vi "RP100 ini.vi"(7 "Error Queue Option":enum16{"Clear Error Queue", "Error Query"}(ring), 8 "error in (no error)":errorcluster, 9 "ID Query? (T)":bool, 10 "Reset? (T)":bool, 11 "VISA resource name":refnum<visa-resource-name>) -> (0 "error out":errorcluster, 3 "VISA resource name out":refnum<visa-resource-name>)   [LabVIEW 2019, in "RP100.lvlib"]
uses:
  RP100.lvlib
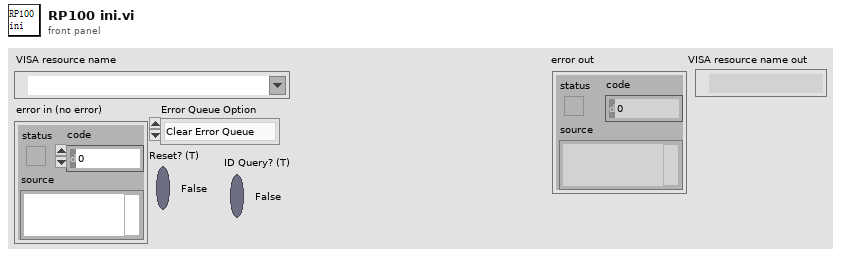
[diagram p1: front panel]
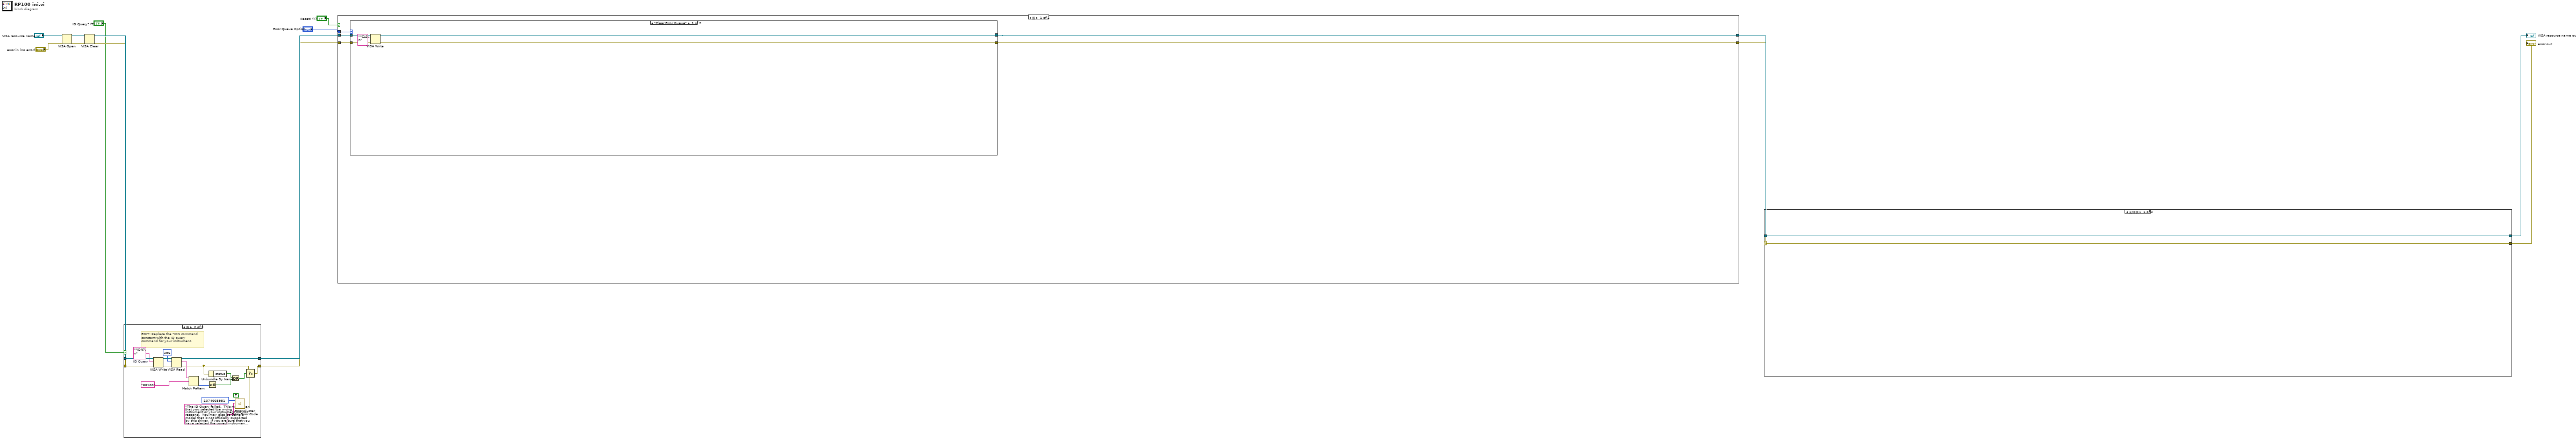
[diagram p0: block diagram]
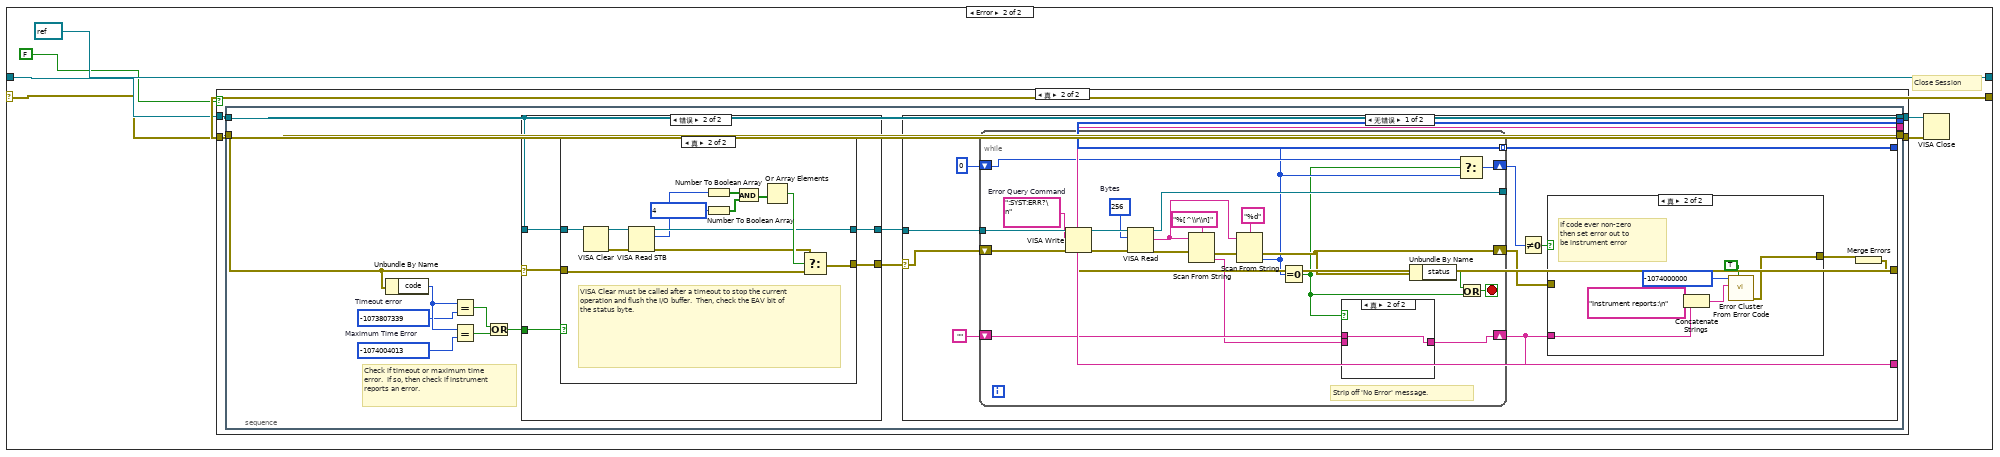
[diagram p2: hidden frame]
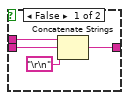
[diagram p7: hidden frame]
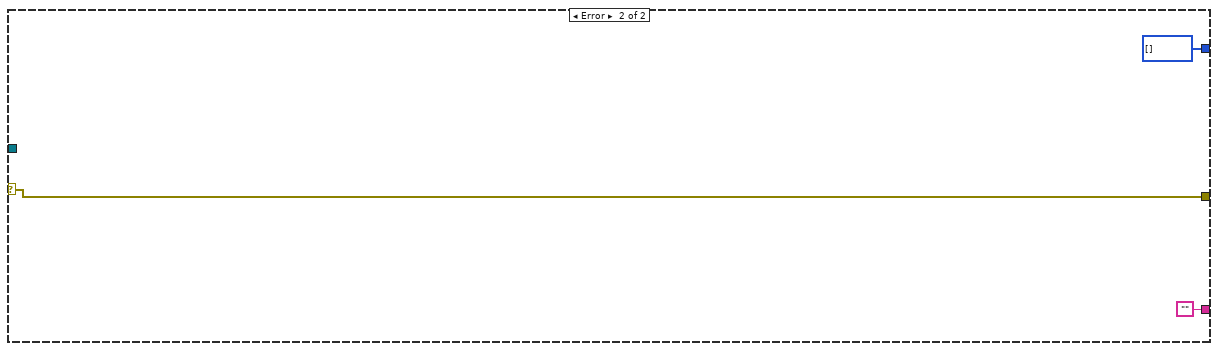
[diagram p8: hidden frame]
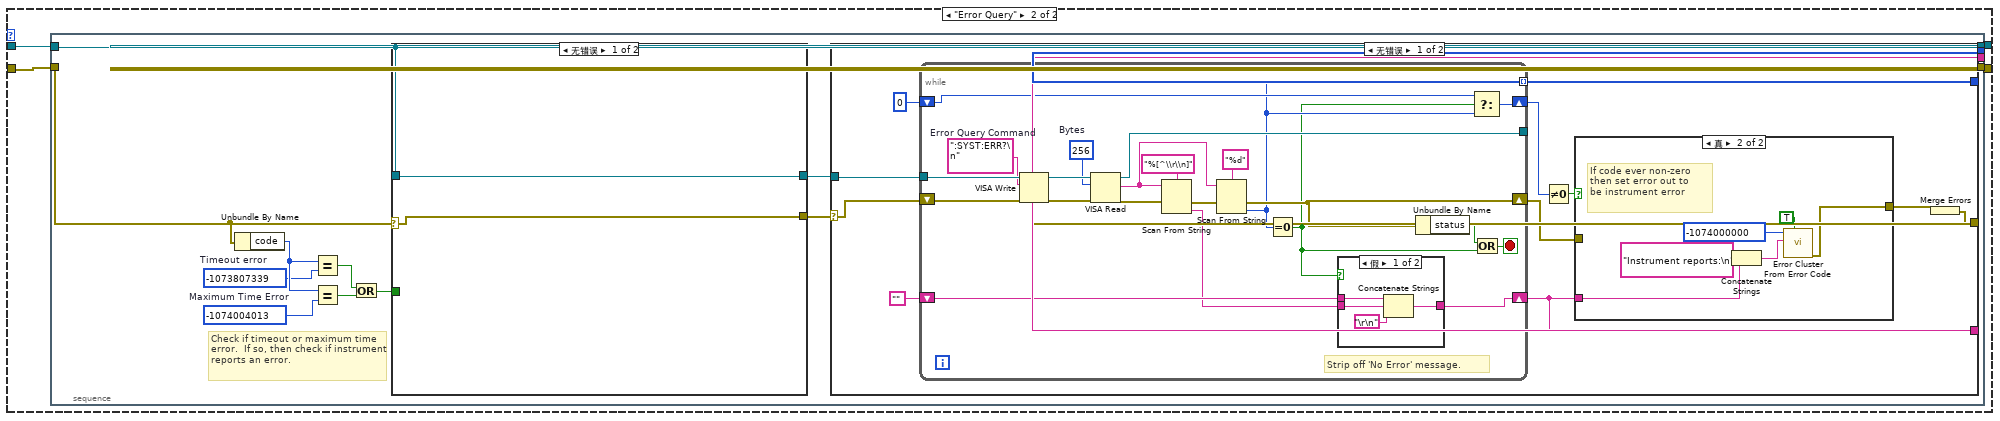
[diagram p9: hidden frame]
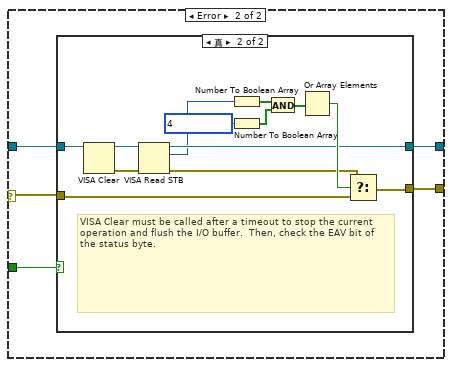
[diagram p10: hidden frame]
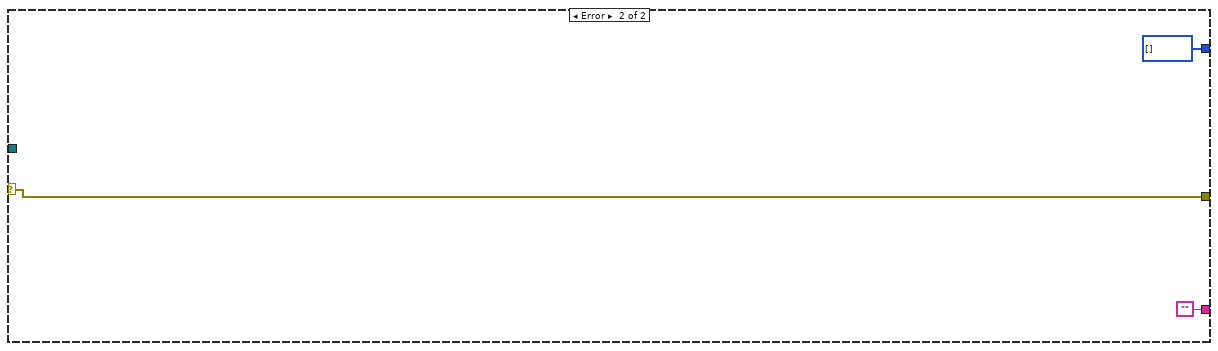
[diagram p14: hidden frame]
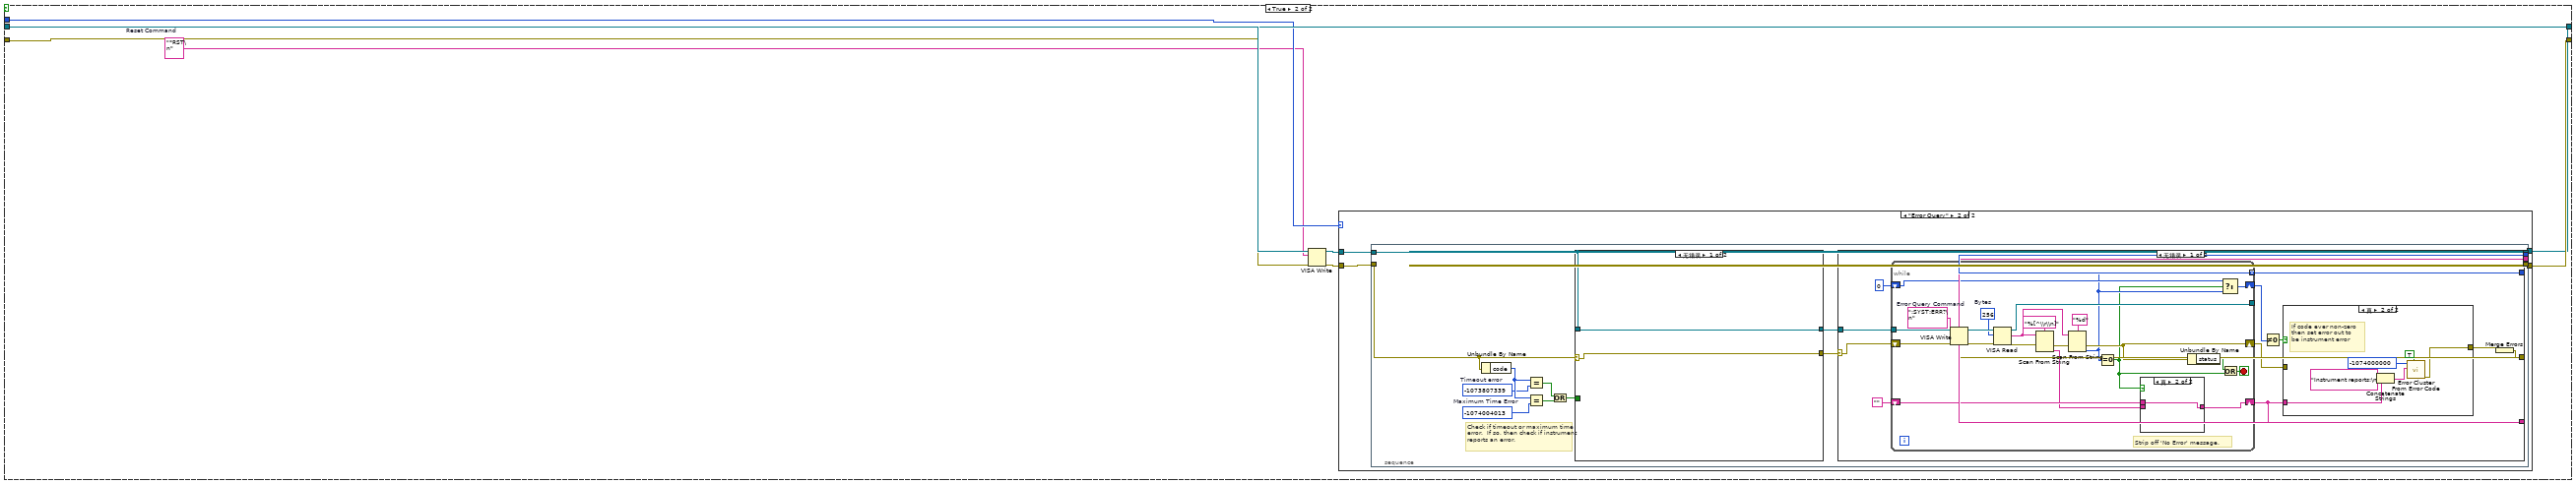
[diagram p15: hidden frame]
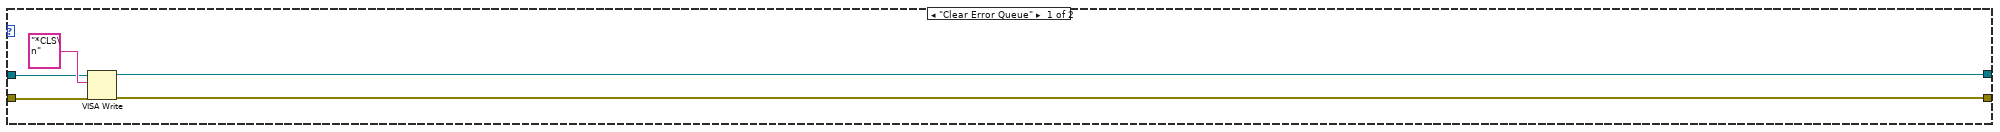
[diagram p16: hidden frame]
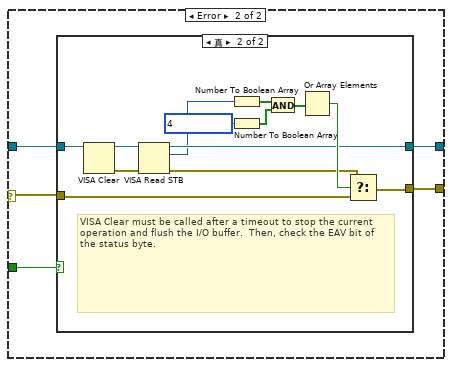
[diagram p17: hidden frame]
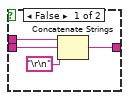
[diagram p20: hidden frame]
diagram:
  n1 = VISA Open(error in (no error)="error in (no error)", VISA resource name="VISA resource name") -> (VISA resource name=w14:refnum<visa-resource-name>, error out=w11:errorcluster)  [unwired: 3 in]
  n2 = VISA Clear(VISA resource name=w14, error in (no error)=w11) -> (VISA resource name out=w13:refnum<visa-resource-name>, error out=w12:errorcluster)
  n3 = case shown="真" "ID Query? (T)" {
    tunnel: [w16 w36] -> w8
    tunnel: [w17 w33] -> w9
    tunnel: w13 -> [w17 w34]
    tunnel: w12 -> [w16 w35]
    frame False {
    }
    frame True {
      w28 = "*IDN?\n"  # ID Query
      # "EDIT: Replace the *IDN command\nconstant with the ID query\ncommand for your instrument."
      n4 = VISA Write(VISA resource name=w34, write buffer=w28, error in (no error)=w35) -> (VISA resource name out=w31:refnum<visa-resource-name>, error out=w30:errorcluster)  [unwired: 1 out]
      n5 = VISA Read(VISA resource name=w31, byte count=u32 256, error in (no error)=w30) -> (VISA resource name out=w33:refnum<visa-resource-name>, read buffer=w32:string, error out=w22:errorcluster)  [unwired: 1 out]
      n6 = Match Pattern(string=w32, regular expression="RP100") -> (offset past match=w23:i32)  [unwired: 1 in, 3 out]
      n7 = Greater Or Equal To 0?(x=w23) -> (x >= 0?=w20:bool)
      n8 = Unbundle By Name(w22) -> ("status"=w21:bool)
      n9 = Or(x=w21, y=w20) -> (x .or. y?=w19:bool)
      n10 = call <vilib>:"Error Cluster From Error Code.vi"("show call chain? (False)"=TRUE, "error message (\"\")"="The ID Query failed.  This may mean that you selected the wrong instrument or your instrument did not respond.  You may also be using a model that is not officially supported by this driver.  If you are sure that you have selected the correct instrument and it is responding, try disabling the ID Query." ("Source (VI Name)"), "error code (0)"=-1074003951 ("Code")) -> ("error out"=w27:errorcluster)  [unwired: 6 in]
      n11 = Select(t=w22, s=w19, f=w27) -> (s? t:f=w36:errorcluster)
    }
  }
  n12 = case shown="假" "Reset? (T)" {
    tunnel: w8 -> [w38 w140]
    tunnel: [w40 w139] -> w4
    tunnel: w9 -> [w39 w141]
    tunnel: [w41 w138] -> w5
    tunnel: "Error Queue Option" -> [w37 w137]
    frame False {
      n13 = case shown="\"Clear Error Queue\"" w37 {
        tunnel: [w43 w50] -> w41
        tunnel: [w44 w49] -> w40
        tunnel: w39 -> [w46 w48]
        tunnel: w38 -> [w45 w47]
        frame "Clear Error Queue" {
          n14 = VISA Write(VISA resource name=w46, write buffer="*CLS\n", error in (no error)=w45) -> (VISA resource name out=w43:refnum<visa-resource-name>, error out=w44:errorcluster)  [unwired: 1 out]
        }
        frame "Error Query" {
          n15 = stacked-sequence {
            tunnel: w48 -> [w63]
            tunnel: [w63] -> w50
            tunnel: [w53] -> _
            tunnel: [w52] -> _
            tunnel: w47 -> [w62]
            tunnel: [w51] -> w49
            frame #0 {
              w58 = -1074004013  # Maximum Time Error
              w56 = -1073807339  # Timeout error
              # "Check if timeout or maximum time error.  If so, then check if instrument reports an error."
              n16 = Unbundle By Name(w62) -> ("code"=w57:i32)
              n17 = Equal?(x=w57, y=w56) -> (x = y?=w60:bool)
              n18 = Equal?(x=w57, y=w58) -> (x = y?=w59:bool)
              n19 = Or(x=w60, y=w59) -> (x .or. y?=w61:bool)
              n20 = case shown="无错误" w62 {
                selector: w62 -> [w64 w68]
                tunnel: w63 -> [w65 w70]
                tunnel: [w65 w69] -> w55
                tunnel: [w64 w67] -> w54
                tunnel: w61 -> [_ w66]
                frame No Error {
                }
                frame Error {
                  n21 = case shown="真" w66 {
                    tunnel: w70 -> [w72 w78]
                    tunnel: [w72 w75] -> w69
                    tunnel: w68 -> [w71 w81]
                    tunnel: [w71 w80] -> w67
                    frame False {
                      # "Error code not a timeout, so best to pass on to user."
                    }
                    frame True {
                      # "VISA Clear must be called after a timeout to stop the current operation and flush the I/O buffer.  Then, check the EAV bit of the status byte."
                      n22 = VISA Clear(VISA resource name=w78) -> (VISA resource name out=w77:refnum<visa-resource-name>, error out=w76:errorcluster)  [unwired: 1 in]
                      n23 = VISA Read STB(8:w76, 11:w77) -> (0:w74:errorcluster, 2:w73:u16, 3:w75:refnum<visa-resource-name>)
                      n24 = Number To Boolean Array(number=w73) -> (Boolean array=w82:bool[])
                      n25 = Number To Boolean Array(number=u8 4) -> (Boolean array=w84:bool[])
                      n26 = And(x=w82, y=w84) -> (x .and. y?=w83:bool[])
                      n27 = Or Array Elements(Boolean array=w83) -> (logical OR=w79:bool)
                      n28 = Select(t=w74, s=w79, f=w81) -> (s? t:f=w80:errorcluster)
                    }
                  }
                }
              }
              n29 = case shown="无错误" w54 {
                selector: w54 -> [w86 w131]
                tunnel: w55 -> [w96 _]
                tunnel: [w94 w131] -> w51
                tunnel: [w89 ""] -> w52
                tunnel: [w88 i32[] []] -> w53
                frame No Error {
                  n30 = while {
                    tunnel: [w125] -> _
                    tunnel: w96 -> [w124]
                    shift-right: [w113] -> w89
                    shift-left: "" -> [w115]
                    shift-right: [w111] -> w90
                    shift-left: 0 -> [w112]
                    shift-right: [w109] -> w87
                    shift-left: w86 -> [w110]
                    tunnel: [w105] -> w88 mode=indexing
                    stop <- w118 stop-if-true
                    w122 = u32 256  # Bytes
                    w120 = ":SYST:ERR?\n"  # Error Query Command
                    # "Strip off 'No Error' message."
                    n31 = VISA Write(VISA resource name=w124, write buffer=w120, error in (no error)=w110) -> (VISA resource name out=w123:refnum<visa-resource-name>, error out=w121:errorcluster)  [unwired: 1 out]
                    n32 = VISA Read(VISA resource name=w123, byte count=w122, error in (no error)=w121) -> (VISA resource name out=w125:refnum<visa-resource-name>, read buffer=w116:string, error out=w108:errorcluster)  [unwired: 1 out]
                    n33 = Scan From String(format string="%[^\\r\\n]", input string=w116, error in=w108) -> (error out=w107:errorcluster, output 1=w114:string)  [unwired: 1 in, 3 out]
                    n34 = Scan From String(format string="%d", input string=w116, error in=w107) -> (error out=w109:errorcluster, output 1=w105:i32)  [unwired: 1 in, 3 out]
                    n35 = Equal To 0?(x=w105) -> (x = 0?=w104:bool)
                    n36 = case shown="假" w104 {
                      tunnel: w115 -> [w129 w130]
                      tunnel: w114 -> [w127 _]
                      tunnel: [w126 w130] -> w113
                      frame False {
                        n37 = Concatenate Strings(w129, w127, "\r\n") -> (w126:string)
                      }
                      frame True {
                      }
                    }
                    n38 = Unbundle By Name(w109) -> ("status"=w106:bool)
                    n39 = Select(t=w112, s=w104, f=w105) -> (s? t:f=w111:i32)
                    n40 = Or(x=w106, y=w104) -> (x .or. y?=w118:bool)
                  }
                  n41 = Not Equal To 0?(x=w90) -> (x != 0?=w92:bool)
                  n42 = case shown="真" w92 {
                    tunnel: w89 -> [_ w102]
                    tunnel: [w97 w98] -> w91
                    tunnel: w87 -> [w97 _]
                    frame False {
                    }
                    frame True {
                      # "If code ever non-zero\nthen set error out to\nbe instrument error"
                      n43 = Concatenate Strings("Instrument reports:\n" ("Source"), w102) -> (w99:string)
                      n44 = call <vilib>:"Error Cluster From Error Code.vi"("show call chain? (False)"=TRUE, "error message (\"\")"=w99, "error code (0)"=-1074000000 ("Code")) -> ("error out"=w98:errorcluster)  [unwired: 1 in, 5 out]
                    }
                  }
                  n45 = Merge Errors(w91) -> (w94:errorcluster)
                }
                frame Error {
                }
              }
            }
          }
        }
      }
    }
    frame True {
      w134 = "*RST\n"  # Reset Command
      n46 = VISA Write(VISA resource name=w141, write buffer=w134, error in (no error)=w140) -> (VISA resource name out=w136:refnum<visa-resource-name>, error out=w135:errorcluster)  [unwired: 1 out]
      n47 = case shown="\"Error Query\"" w137 {
        tunnel: [w142 w150] -> w138
        tunnel: [w145 w149] -> w139
        tunnel: w135 -> [w146 w147]
        tunnel: w136 -> [w143 w148]
        frame "Clear Error Queue" {
          n48 = VISA Write(VISA resource name=w143, write buffer="*CLS\n", error in (no error)=w146) -> (VISA resource name out=w142:refnum<visa-resource-name>, error out=w145:errorcluster)  [unwired: 1 out]
        }
        frame "Error Query" {
          n49 = stacked-sequence {
            tunnel: w148 -> [w163]
            tunnel: [w163] -> w150
            tunnel: [w153] -> _
            tunnel: [w152] -> _
            tunnel: w147 -> [w162]
            tunnel: [w151] -> w149
            frame #0 {
              w158 = -1074004013  # Maximum Time Error
              w156 = -1073807339  # Timeout error
              # "Check if timeout or maximum time error.  If so, then check if instrument reports an error."
              n50 = Unbundle By Name(w162) -> ("code"=w157:i32)
              n51 = Equal?(x=w157, y=w156) -> (x = y?=w160:bool)
              n52 = Equal?(x=w157, y=w158) -> (x = y?=w159:bool)
              n53 = Or(x=w160, y=w159) -> (x .or. y?=w161:bool)
              n54 = case shown="无错误" w162 {
                selector: w162 -> [w164 w168]
                tunnel: w163 -> [w165 w170]
                tunnel: [w165 w169] -> w155
                tunnel: [w164 w167] -> w154
                tunnel: w161 -> [_ w166]
                frame No Error {
                }
                frame Error {
                  n55 = case shown="真" w166 {
                    tunnel: w170 -> [w172 w178]
                    tunnel: [w172 w175] -> w169
                    tunnel: w168 -> [w171 w181]
                    tunnel: [w171 w180] -> w167
                    frame False {
                      # "Error code not a timeout, so best to pass on to user."
                    }
                    frame True {
                      # "VISA Clear must be called after a timeout to stop the current operation and flush the I/O buffer.  Then, check the EAV bit of the status byte."
                      n56 = VISA Clear(VISA resource name=w178) -> (VISA resource name out=w177:refnum<visa-resource-name>, error out=w176:errorcluster)  [unwired: 1 in]
                      n57 = VISA Read STB(8:w176, 11:w177) -> (0:w174:errorcluster, 2:w173:u16, 3:w175:refnum<visa-resource-name>)
                      n58 = Number To Boolean Array(number=w173) -> (Boolean array=w182:bool[])
                      n59 = Number To Boolean Array(number=u8 4) -> (Boolean array=w184:bool[])
                      n60 = And(x=w182, y=w184) -> (x .and. y?=w183:bool[])
                      n61 = Or Array Elements(Boolean array=w183) -> (logical OR=w179:bool)
                      n62 = Select(t=w174, s=w179, f=w181) -> (s? t:f=w180:errorcluster)
                    }
                  }
                }
              }
              n63 = case shown="无错误" w154 {
                selector: w154 -> [w186 w231]
                tunnel: w155 -> [w196 _]
                tunnel: [w194 w231] -> w151
                tunnel: [w189 ""] -> w152
                tunnel: [w188 i32[] []] -> w153
                frame No Error {
                  n64 = while {
                    tunnel: [w225] -> _
                    tunnel: w196 -> [w224]
                    shift-right: [w213] -> w189
                    shift-left: "" -> [w215]
                    shift-right: [w211] -> w190
                    shift-left: 0 -> [w212]
                    shift-right: [w209] -> w187
                    shift-left: w186 -> [w210]
                    tunnel: [w205] -> w188 mode=indexing
                    stop <- w218 stop-if-true
                    w222 = u32 256  # Bytes
                    w220 = ":SYST:ERR?\n"  # Error Query Command
                    # "Strip off 'No Error' message."
                    n65 = VISA Write(VISA resource name=w224, write buffer=w220, error in (no error)=w210) -> (VISA resource name out=w223:refnum<visa-resource-name>, error out=w221:errorcluster)  [unwired: 1 out]
                    n66 = VISA Read(VISA resource name=w223, byte count=w222, error in (no error)=w221) -> (VISA resource name out=w225:refnum<visa-resource-name>, read buffer=w216:string, error out=w208:errorcluster)  [unwired: 1 out]
                    n67 = Scan From String(format string="%[^\\r\\n]", input string=w216, error in=w208) -> (error out=w207:errorcluster, output 1=w214:string)  [unwired: 1 in, 3 out]
                    n68 = Scan From String(format string="%d", input string=w216, error in=w207) -> (error out=w209:errorcluster, output 1=w205:i32)  [unwired: 1 in, 3 out]
                    n69 = Equal To 0?(x=w205) -> (x = 0?=w204:bool)
                    n70 = case shown="真" w204 {
                      tunnel: w215 -> [w229 w230]
                      tunnel: w214 -> [w227 _]
                      tunnel: [w226 w230] -> w213
                      frame False {
                        n71 = Concatenate Strings(w229, w227, "\r\n") -> (w226:string)
                      }
                      frame True {
                      }
                    }
                    n72 = Unbundle By Name(w209) -> ("status"=w206:bool)
                    n73 = Select(t=w212, s=w204, f=w205) -> (s? t:f=w211:i32)
                    n74 = Or(x=w206, y=w204) -> (x .or. y?=w218:bool)
                  }
                  n75 = Not Equal To 0?(x=w190) -> (x != 0?=w192:bool)
                  n76 = case shown="真" w192 {
                    tunnel: w189 -> [_ w202]
                    tunnel: [w197 w198] -> w191
                    tunnel: w187 -> [w197 _]
                    frame False {
                    }
                    frame True {
                      # "If code ever non-zero\nthen set error out to\nbe instrument error"
                      n77 = Concatenate Strings("Instrument reports:\n" ("Source"), w202) -> (w199:string)
                      n78 = call <vilib>:"Error Cluster From Error Code.vi"("show call chain? (False)"=TRUE, "error message (\"\")"=w199, "error code (0)"=-1074000000 ("Code")) -> ("error out"=w198:errorcluster)  [unwired: 1 in, 5 out]
                    }
                  }
                  n79 = Merge Errors(w191) -> (w194:errorcluster)
                }
                frame Error {
                }
              }
            }
          }
        }
      }
    }
  }
  n80 = case shown="无错误" w4 {
    selector: w4 -> [w234 w240]
    tunnel: w5 -> [w235 w241]
    tunnel: [w235 refnum<visa-resource-name> refnum ("VISA resource name out")] -> w2
    tunnel: [w234 w242] -> w3
    frame No Error {
    }
    frame Error {
      # "Close Session"
      n81 = case shown="真" FALSE ("Query For SCPI Errors? (T)") {
        tunnel: w241 -> [w244 w248]
        tunnel: w240 -> [w243 w247]
        tunnel: [w243 w246] -> w236
        tunnel: [w244 w245] -> w237
        frame False {
        }
        frame True {
          n82 = stacked-sequence {
            tunnel: w248 -> [w261]
            tunnel: [w261] -> w245
            tunnel: [w251] -> _
            tunnel: [w250] -> _
            tunnel: w247 -> [w260]
            tunnel: [w249] -> w246
            frame #0 {
              w256 = -1074004013  # Maximum Time Error
              w254 = -1073807339  # Timeout error
              # "Check if timeout or maximum time error.  If so, then check if instrument reports an error."
              n83 = Unbundle By Name(w260) -> ("code"=w255:i32)
              n84 = Equal?(x=w255, y=w254) -> (x = y?=w258:bool)
              n85 = Equal?(x=w255, y=w256) -> (x = y?=w257:bool)
              n86 = Or(x=w258, y=w257) -> (x .or. y?=w259:bool)
              n87 = case shown="错误" w260 {
                selector: w260 -> [w262 w266]
                tunnel: w261 -> [w263 w268]
                tunnel: [w263 w267] -> w253
                tunnel: [w262 w265] -> w252
                tunnel: w259 -> [_ w264]
                frame No Error {
                }
                frame Error {
                  n88 = case shown="真" w264 {
                    tunnel: w268 -> [w270 w276]
                    tunnel: [w270 w273] -> w267
                    tunnel: w266 -> [w269 w279]
                    tunnel: [w269 w278] -> w265
                    frame False {
                      # "Error code not a timeout, so best to pass on to user."
                    }
                    frame True {
                      # "VISA Clear must be called after a timeout to stop the current operation and flush the I/O buffer.  Then, check the EAV bit of the status byte."
                      n89 = VISA Clear(VISA resource name=w276) -> (VISA resource name out=w275:refnum<visa-resource-name>, error out=w274:errorcluster)  [unwired: 1 in]
                      n90 = VISA Read STB(8:w274, 11:w275) -> (0:w272:errorcluster, 2:w271:u16, 3:w273:refnum<visa-resource-name>)
                      n91 = Number To Boolean Array(number=w271) -> (Boolean array=w280:bool[])
                      n92 = Number To Boolean Array(number=u8 4) -> (Boolean array=w282:bool[])
                      n93 = And(x=w280, y=w282) -> (x .and. y?=w281:bool[])
                      n94 = Or Array Elements(Boolean array=w281) -> (logical OR=w277:bool)
                      n95 = Select(t=w272, s=w277, f=w279) -> (s? t:f=w278:errorcluster)
                    }
                  }
                }
              }
              n96 = case shown="无错误" w252 {
                selector: w252 -> [w284 w329]
                tunnel: w253 -> [w294 _]
                tunnel: [w292 w329] -> w249
                tunnel: [w287 ""] -> w250
                tunnel: [w286 i32[] []] -> w251
                frame No Error {
                  n97 = while {
                    tunnel: [w323] -> _
                    tunnel: w294 -> [w322]
                    shift-right: [w311] -> w287
                    shift-left: "" -> [w313]
                    shift-right: [w309] -> w288
                    shift-left: 0 -> [w310]
                    shift-right: [w307] -> w285
                    shift-left: w284 -> [w308]
                    tunnel: [w303] -> w286 mode=indexing
                    stop <- w316 stop-if-true
                    w320 = u32 256  # Bytes
                    w318 = ":SYST:ERR?\n"  # Error Query Command
                    # "Strip off 'No Error' message."
                    n98 = VISA Write(VISA resource name=w322, write buffer=w318, error in (no error)=w308) -> (VISA resource name out=w321:refnum<visa-resource-name>, error out=w319:errorcluster)  [unwired: 1 out]
                    n99 = VISA Read(VISA resource name=w321, byte count=w320, error in (no error)=w319) -> (VISA resource name out=w323:refnum<visa-resource-name>, read buffer=w314:string, error out=w306:errorcluster)  [unwired: 1 out]
                    n100 = Scan From String(format string="%[^\\r\\n]", input string=w314, error in=w306) -> (error out=w305:errorcluster, output 1=w312:string)  [unwired: 1 in, 3 out]
                    n101 = Scan From String(format string="%d", input string=w314, error in=w305) -> (error out=w307:errorcluster, output 1=w303:i32)  [unwired: 1 in, 3 out]
                    n102 = Equal To 0?(x=w303) -> (x = 0?=w302:bool)
                    n103 = case shown="真" w302 {
                      tunnel: w313 -> [w327 w328]
                      tunnel: w312 -> [w325 _]
                      tunnel: [w324 w328] -> w311
                      frame False {
                        n104 = Concatenate Strings(w327, w325, "\r\n") -> (w324:string)
                      }
                      frame True {
                      }
                    }
                    n105 = Unbundle By Name(w307) -> ("status"=w304:bool)
                    n106 = Select(t=w310, s=w302, f=w303) -> (s? t:f=w309:i32)
                    n107 = Or(x=w304, y=w302) -> (x .or. y?=w316:bool)
                  }
                  n108 = Not Equal To 0?(x=w288) -> (x != 0?=w290:bool)
                  n109 = case shown="真" w290 {
                    tunnel: w287 -> [_ w300]
                    tunnel: [w295 w296] -> w289
                    tunnel: w285 -> [w295 _]
                    frame False {
                    }
                    frame True {
                      # "If code ever non-zero\nthen set error out to\nbe instrument error"
                      n110 = Concatenate Strings("Instrument reports:\n" ("Source"), w300) -> (w297:string)
                      n111 = call <vilib>:"Error Cluster From Error Code.vi"("show call chain? (False)"=TRUE, "error message (\"\")"=w297, "error code (0)"=-1074000000 ("Code")) -> ("error out"=w296:errorcluster)  [unwired: 1 in, 5 out]
                    }
                  }
                  n112 = Merge Errors(w289) -> (w292:errorcluster)
                }
                frame Error {
                }
              }
            }
          }
        }
      }
      n113 = VISA Close(VISA resource name=w237, error in (no error)=w236) -> (error out=w242:errorcluster)
    }
  }
  "error out" <- w3
  "VISA resource name out" <- w2
